vi "Initialize Data Attributes.vi"(8 "error in (no error)":errorcluster) -> (0 "error out":errorcluster, 3 "Data.lvclass":refnum<class "Data.lvclass">)   [LabVIEW 2017, in "Data.lvclass"]
uses:
  <vilib>/addons/_NISVFA/_Shared subVIs/Data Objects/Data/Data.lvclass
  <vilib>/addons/_NISVFA/_Shared subVIs/Data Objects/Data/Data.lvclass/Data.ctl
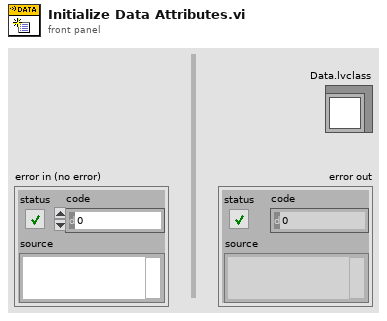
[diagram p1: front panel]
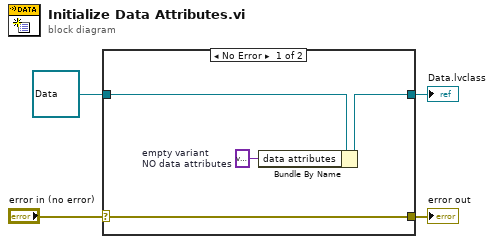
[diagram p0: block diagram]
diagram:
  n1 = case shown="No Error" "error in (no error)" {
    selector: "error in (no error)" -> [w5 w10]
    tunnel: refnum<class "Data.lvclass"> refnum ("Data.lvclass") -> [w8 w9]
    tunnel: [w7 w9] -> w3
    tunnel: [w5 w10] -> w1
    frame No Error {
      w6 = variant  # empty variant NO data attributes
      n2 = Bundle By Name(cluster=w8, "data attributes"=w6) -> (w7:refnum<class "Data.lvclass">)
    }
    frame Error {
    }
  }
  "Data.lvclass" <- w3
  "error out" <- w1
